vi "CalculateCapacitance.vi"(9 "Frequency (Hz)":dbl, 10 "Theta (Phase)":dbl, 11 "Z (impedance)":dbl) -> (2 "Cs [pF]":dbl, 3 "Cp [pF]":dbl)   [LabVIEW 2016]
panel:
  out "Rs [Ohm]":dbl
  out "Rp [Ohm]":dbl
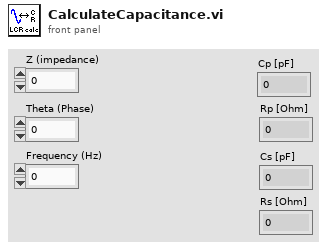
[diagram p1: front panel]
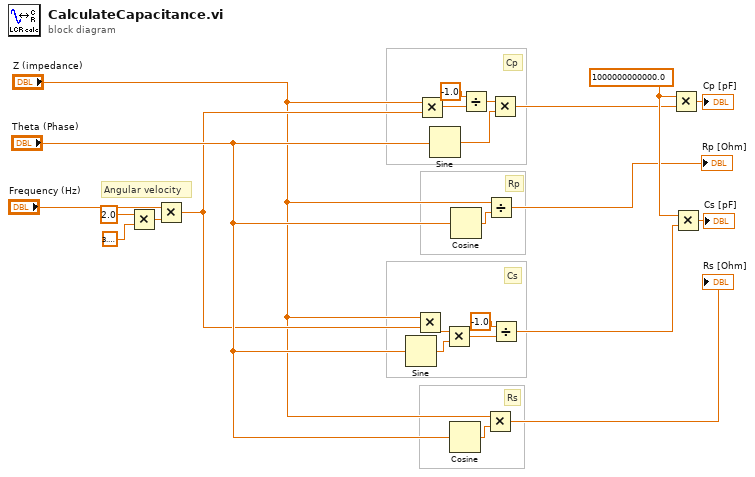
[diagram p0: block diagram]
diagram:
  w22 = 1000000000000.0 ("y")
  # "Cp"
  # "Angular velocity"
  # "Rp"
  # "Cs"
  # "Rs"
  n1 = Multiply(x=2.0, y=3.141592653589793) -> (x*y=w16:dbl)
  n2 = Multiply(x="Frequency (Hz)", y=w16) -> (x*y=w3:dbl)
  n3 = Sine(x="Theta (Phase)") -> (sin(x)=w13:dbl)
  n4 = Multiply(x="Z (impedance)", y=w3) -> (x*y=w14:dbl)
  n5 = Multiply(x="Z (impedance)", y=w3) -> (x*y=w4:dbl)
  n6 = Sine(x="Theta (Phase)") -> (sin(x)=w6:dbl)
  n7 = Multiply(x=w14, y=w13) -> (x*y=w12:dbl)
  n8 = Cosine(x="Theta (Phase)") -> (cos(x)=w21:dbl)
  n9 = Cosine(x="Theta (Phase)") -> (cos(x)=w10:dbl)
  n10 = Divide(x=-1.0, y=w4) -> (x/y=w7:dbl)
  n11 = Multiply(x="Z (impedance)", y=w21) -> (x*y=→"Rs [Ohm]":dbl)
  n12 = Divide(x="Z (impedance)", y=w10) -> (x/y=→"Rp [Ohm]":dbl)
  n13 = Multiply(x=w7, y=w6) -> (x*y=w1:dbl)
  n14 = Divide(x=-1.0, y=w12) -> (x/y=w11:dbl)
  n15 = Multiply(x=w22, y=w1) -> (x*y=→"Cp [pF]":dbl)
  n16 = Multiply(x=w22, y=w11) -> (x*y=→"Cs [pF]":dbl)
